vi "PID Loop Property.vi"(2 "error in (no error)":errorcluster, 3 "LBCB Number":T2) -> (0 "error out":errorcluster)   [LabVIEW 2009]
uses:
  lib/Data Access Objects/Metadata/LBCB Number.ctl
  lib/Data Access Objects/Metadata/Actuator Point.ctl
  Update Actions.ctl
  lib/Data Access Objects/Application/Number Of LBCBs.ctl
  lib/Data Access Objects/Metadata/Persistant DAO Actions.ctl
panel:
  out "L2 Default P Gain":T1
  out "L2 Default I Gain":T1
  out "L1 Default P Gain":T1
  out "L1 Default I Gain":T1
  in  "P Gain":dbl[](array[numeric])=[0.02, 0.02, 0.02, 0.02, 0.02, 0.02] caption="Proportional Gain (suggested value 0)"
  in  "Cancel":bool
  in  "OK":bool
  in  "I Gain":dbl[](array[numeric])=[0.02, 0.02, 0.02, 0.02, 0.02, 0.02] caption="Integrator Gain"
  # "Middle Feedback Loop Properties (PI Control)"
  # "Actuator X1"
  # "Actuator X2"
  # "Actuator Y1"
  # "Actuator Z1"
  # "Actuator Z2"
  # "Actuator Z3"
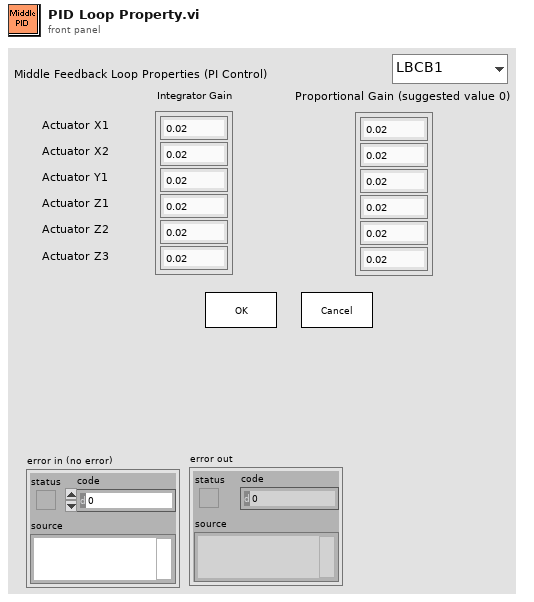
[diagram p1: front panel]
types:
  T1 = typedef "Actuator Point.ctl" = cluster{"X1":dbl, "X2":dbl, "Y1":dbl, "Z1":dbl, "Z2":dbl, "Z3":dbl}
  T2 = typedef "LBCB Number.ctl" = enum16{"LBCB1", "LBCB2"}
  T3 = typedef "Update Actions.ctl" = enum16{"Update", "Exit"}
  T4 = enum8{"Enabled", "Disabled", "Disabled and Grayed Out"}
  T5 = typedef "Number Of LBCBs.ctl" = enum16{"1", "2"}
  T6 = typedef "Persistant DAO Actions.ctl" = enum16{"Init", "Get", "Set", "Load", "Save"}
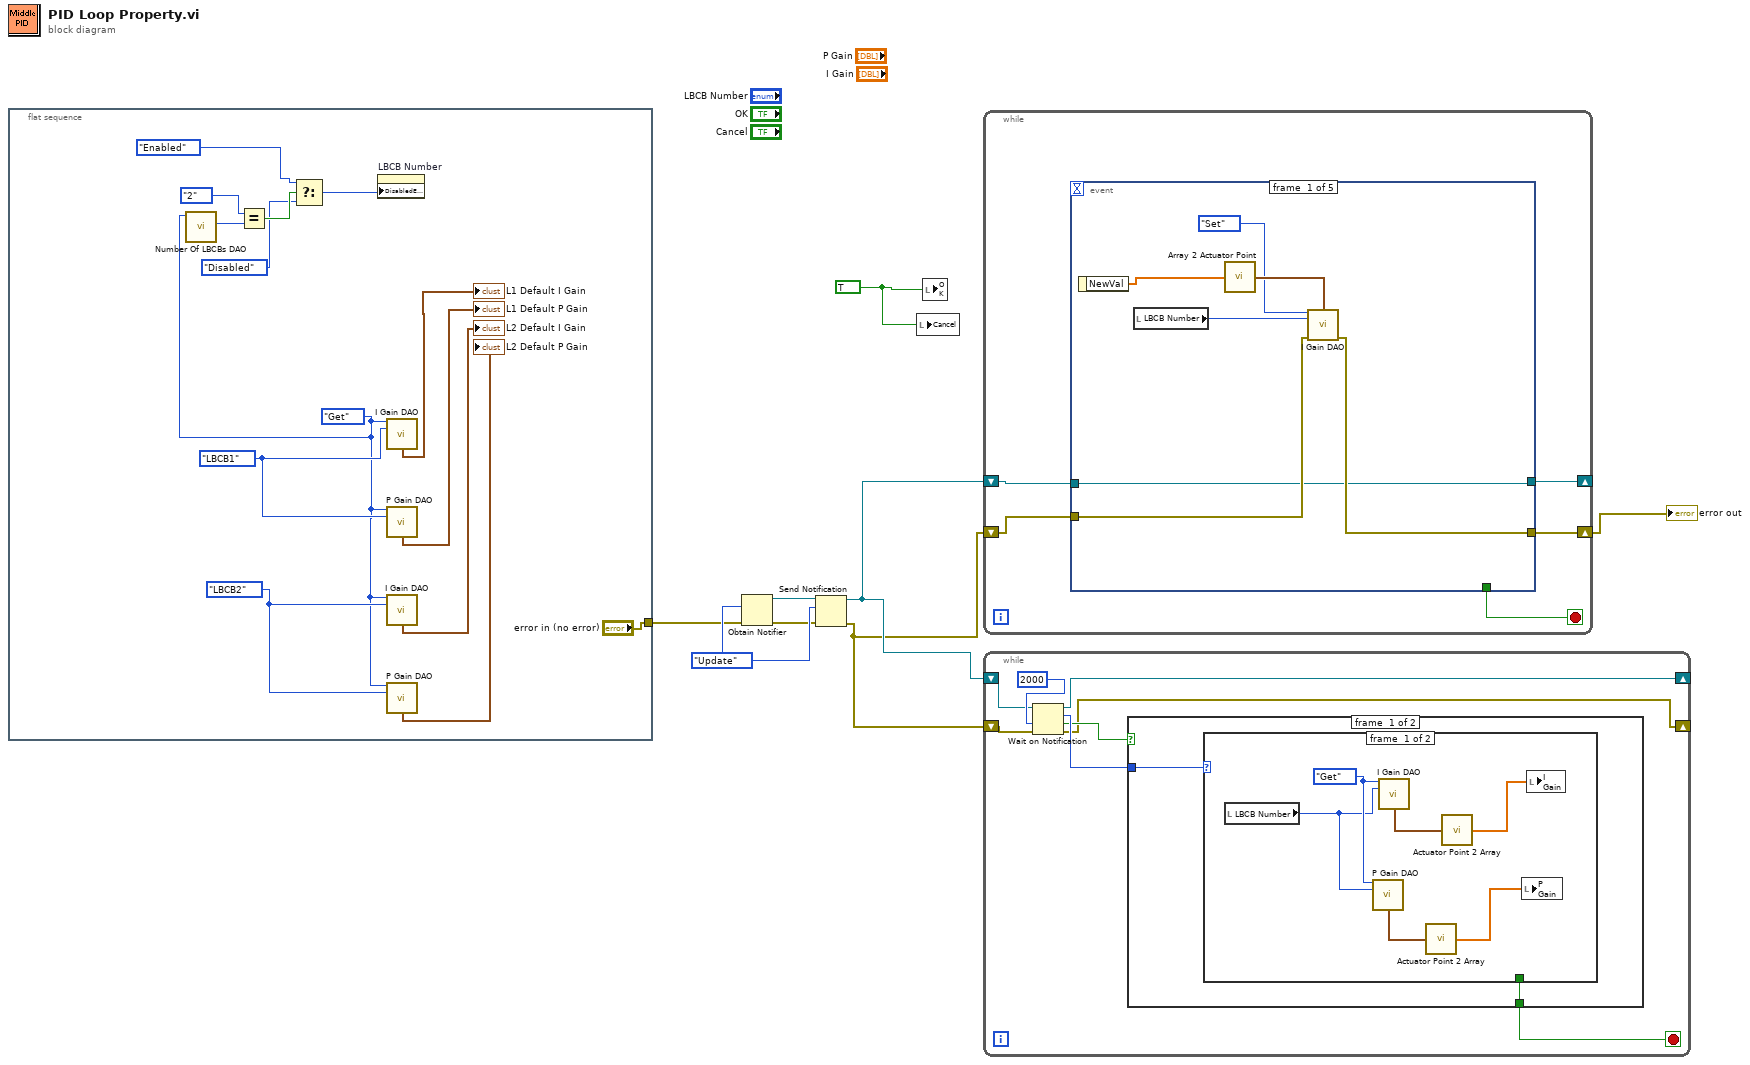
[diagram p0: block diagram]
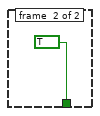
[diagram p2: hidden frame]
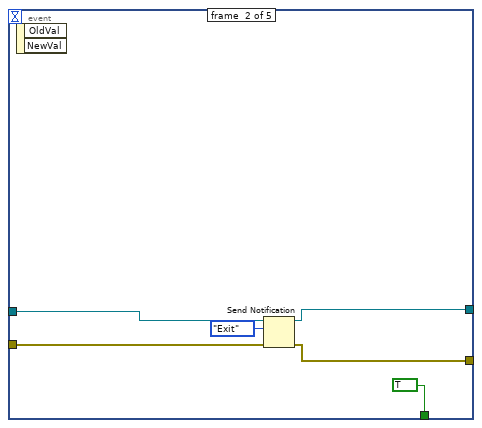
[diagram p4: hidden frame]
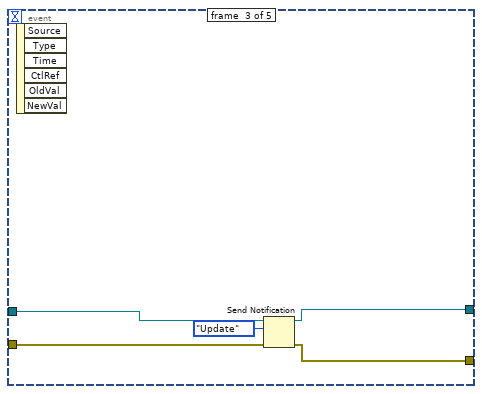
[diagram p5: hidden frame]
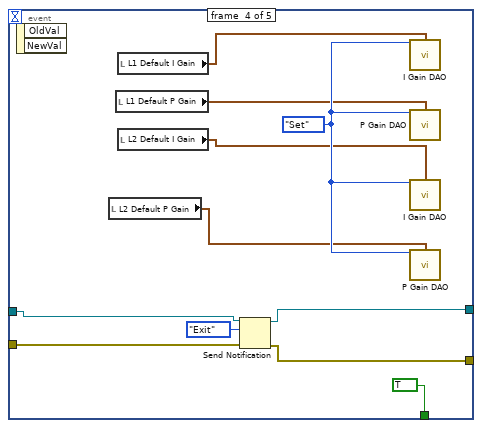
[diagram p6: hidden frame]
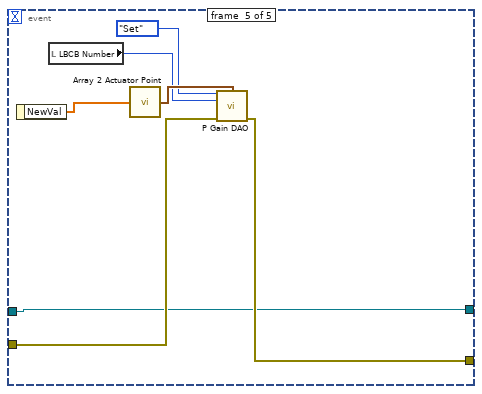
[diagram p7: hidden frame]
diagram:
  w1 = TRUE ("OK")
  w8 = Update_Actions."Update" ("Update Actions")
  n1 = flat-sequence {
    tunnel: ["error in (no error)"] -> w5
    frame #0 {
      w20 = LBCB_Number."LBCB2" ("LBCB Number")
      w21 = LBCB_Number."LBCB1" ("LBCB Number")
      w10 = Persistant_DAO_Actions."Get" ("I Gain Actions")
      n2 = call "Number Of LBCBs DAO.vi"("Actions"=w10) -> ("Number of\nLBCBs Out"=w15:T5)  [unwired: 8 in, 2 out]
      n3 = Equal?(x=Number_Of_LBCBs."2", y=w15) -> (x = y?=w13:bool)
      n4 = Select(t=T4."Enabled" ("Disabled"), s=w13, f=T4."Disabled") -> (s? t:f=w9:T4)
      n5 = property on="LBCB Number" class="Enum (strict)"("DisabledEnum"=w9) -> ()  [unwired: 2 in, 2 out]
      n6 = call "I Gain DAO.vi"("I Gain Actions"=w10, "LBCB Number"=w21) -> ("I Gain"=→"L1 Default I Gain":T1)  [unwired: 3 in, 10 out]
      n7 = call "P Gain DAO.vi"("P Gain Actions"=w10, "LBCB Number"=w21) -> ("P Gain"=→"L1 Default P Gain":T1)  [unwired: 3 in, 10 out]
      n8 = call "I Gain DAO.vi"("I Gain Actions"=w10, "LBCB Number"=w20) -> ("I Gain"=→"L2 Default I Gain":T1)  [unwired: 3 in, 10 out]
      n9 = call "P Gain DAO.vi"("P Gain Actions"=w10, "LBCB Number"=w20) -> ("P Gain"=→"L2 Default P Gain":T1)  [unwired: 3 in, 10 out]
    }
  }
  n10 = Obtain Notifier(notification data type=w8, error in (no error)=w5) -> (notifier out=w7:refnum<notifier>, error out=w6:errorcluster)  [unwired: 1 in, 2 out]
  n11 = Send Notification(notification=w8, notifier=w7, error in (no error)=w6) -> (notifier out=w4:refnum<notifier>, error out=w3:errorcluster)
  n12 = local write "Cancel"(w1) -> ()
  n13 = local write "OK"(w1) -> ()
  n14 = while {
    shift-right: [w24] -> _
    shift-left: w4 -> [w26]
    shift-right: [w23] -> w2
    shift-left: w3 -> [w25]
    stop <- w27 stop-if-true
    n15 = event shown="[2] \"LBCB Number\": Value Change" {
      selector: _ -> [_ _ _ _ _]
      dyn-events: _ -> [_ _ _ _ _]
      timeout: _ -> [_ _ _ _ _]
      tunnel: [_ TRUE _ TRUE _] -> w27
      tunnel: w26 -> [w28 w39 w45 w49 w57]
      tunnel: w25 -> [w30 w38 w44 w48 w59]
      tunnel: [w28 w37 w43 w47 w57] -> w24
      tunnel: [w29 w36 w42 w46 w58] -> w23
      event #0 {
        n16 = event-data() -> ("NewVal"=w34:dbl[])  [unwired: 1 out]
        n17 = local read "LBCB Number"() -> (w31:T2)
        n18 = call "Array 2 Actuator Point.vi"("Array"=w34) -> ("Actuator Point"=w33:T1)
        n19 = call "I Gain DAO.vi"("I Gain Actions"=Persistant_DAO_Actions."Set", "I Gain In"=w33, "LBCB Number"=w31, "error in (no error)"=w30) -> ("error out"=w29:errorcluster)  [unwired: 1 in, 10 out]
      }
      event #1 {
        n20 = event-data() -> ()  [unwired: 3 out]
        n21 = Send Notification(notification=Update_Actions."Exit", notifier=w39, error in (no error)=w38) -> (notifier out=w37:refnum<notifier>, error out=w36:errorcluster)
      }
      event #2 {
        n22 = event-data() -> ()  [unwired: 7 out]
        n23 = Send Notification(notification=Update_Actions."Update", notifier=w45, error in (no error)=w44) -> (notifier out=w43:refnum<notifier>, error out=w42:errorcluster)
      }
      event #3 {
        w55 = Persistant_DAO_Actions."Set" ("I Gain Actions")
        n24 = event-data() -> ()  [unwired: 3 out]
        n25 = local read "L2 Default P Gain"() -> (w51:T1)
        n26 = local read "L1 Default P Gain"() -> (w53:T1)
        n27 = local read "L1 Default I Gain"() -> (w54:T1)
        n28 = local read "L2 Default I Gain"() -> (w52:T1)
        n29 = Send Notification(notification=Update_Actions."Exit", notifier=w49, error in (no error)=w48) -> (notifier out=w47:refnum<notifier>, error out=w46:errorcluster)
        n30 = call "I Gain DAO.vi"("I Gain Actions"=w55, "I Gain In"=w54) -> ()  [unwired: 3 in, 11 out]
        n31 = call "P Gain DAO.vi"("P Gain Actions"=w55, "P Gain In"=w53) -> ()  [unwired: 3 in, 11 out]
        n32 = call "I Gain DAO.vi"("I Gain Actions"=w55, "I Gain In"=w52) -> ()  [unwired: 3 in, 11 out]
        n33 = call "P Gain DAO.vi"("P Gain Actions"=w55, "P Gain In"=w51) -> ()  [unwired: 3 in, 11 out]
      }
      event #4 {
        n34 = event-data() -> ("NewVal"=w63:dbl[])  [unwired: 1 out]
        n35 = local read "LBCB Number"() -> (w60:T2)
        n36 = call "Array 2 Actuator Point.vi"("Array"=w63) -> ("Actuator Point"=w62:T1)
        n37 = call "P Gain DAO.vi"("P Gain Actions"=Persistant_DAO_Actions."Set", "P Gain In"=w62, "LBCB Number"=w60, "error in (no error)"=w59) -> ("error out"=w58:errorcluster)  [unwired: 1 in, 10 out]
      }
    }
  }
  "error out" <- w2
  n38 = while {
    shift-right: [w66] -> _
    shift-left: w4 -> [w70]
    shift-right: [w65] -> _
    shift-left: w3 -> [w69]
    stop <- w64 stop-if-true
    n39 = Wait on Notification(notifier=w70, timeout in ms (-1)=2000, error in (no error)=w69) -> (notifier out=w66:refnum<notifier>, notification=w68:T3, timed out?=w67:bool, error out=w65:errorcluster)  [unwired: 1 out]
    n40 = case shown="False" w67 {
      tunnel: w68 -> [w73 _]
      tunnel: [w72 _] -> w64
      frame #0 {
        n41 = case shown="\"Exit\"" w73 {
          tunnel: [_ TRUE] -> w72
          frame #0 {
            w75 = Persistant_DAO_Actions."Get" ("I Gain Actions")
            n42 = local read "LBCB Number"() -> (w74:T2)
            n43 = call "P Gain DAO.vi"("P Gain Actions"=w75, "LBCB Number"=w74) -> ("P Gain"=w79:T1)  [unwired: 3 in, 10 out]
            n44 = call "I Gain DAO.vi"("I Gain Actions"=w75, "LBCB Number"=w74) -> ("I Gain"=w78:T1)  [unwired: 3 in, 10 out]
            n45 = call "Actuator Point 2 Array.vi"("Actuator Point"=w79) -> ("Array"=w77:dbl[])
            n46 = call "Actuator Point 2 Array.vi"("Actuator Point"=w78) -> ("Array"=w76:dbl[])
            n47 = local write "P Gain"(w77) -> ()
            n48 = local write "I Gain"(w76) -> ()
          }
          frame #1 {
          }
        }
      }
      frame #1 {
      }
    }
  }
